vi "Find Selected CSVs From List.vi"(9 "Sel.ItemNames":i32[](array[numeric]), 11 "ListBox Tests":T1) -> (3 "Selected CSVs":path[](array[path]))   [LabVIEW 2011]
uses:
  Controls/ListBox Test Record.ctl
  <userlib>/_OpenG.lib/array/array.llb/Delete Elements from 1D Array (Path)__ogtk.vi
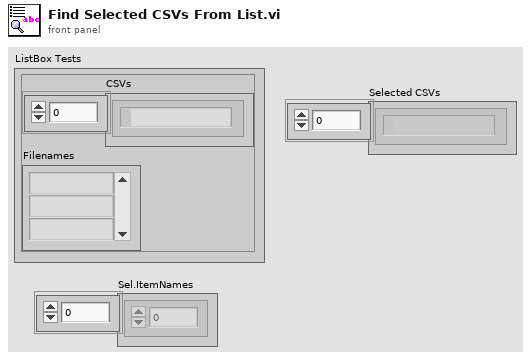
[diagram p1: front panel]
types:
  T1 = typedef "ListBox Test Record.ctl" = cluster{"CSVs":path[], "Filenames":string[]}
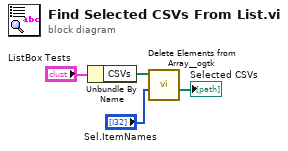
[diagram p0: block diagram]
diagram:
  n1 = Unbundle By Name("ListBox Tests") -> ("CSVs"=w3:path[])
  n2 = call-poly <userlib>:"Delete Elements from Array__ogtk.vi"("indices"="Sel.ItemNames", "array"=w3) -> ("deleted elements"=→"Selected CSVs":path[])  [unwired: 8 in, 1 out]
